vi "CoCreateGUID.vi"(8 "error in (no error)":errorcluster) -> (0 "error out":errorcluster, 2 "GUID":u8[](array[numeric]) format="%x", 4 "GUID string":string)   [LabVIEW 2017]
uses:
  ole32.dll
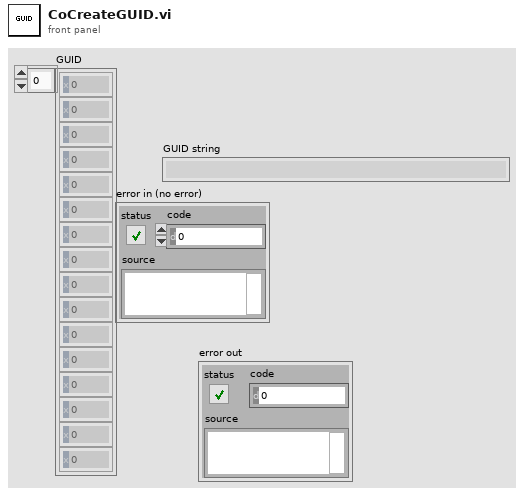
[diagram p1: front panel]
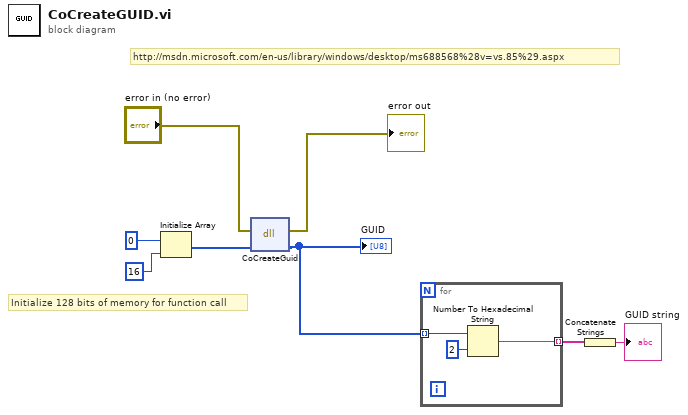
[diagram p0: block diagram]
diagram:
  # "http://msdn.microsoft.com/en-us/library/windows/desktop/ms688568%28v=vs.85%29.aspx"
  # "Initialize 128 bits of memory for function call"
  n1 = Initialize Array(u8 0 ("element"), 16 ("dimension size")) -> (w2:u8[])
  n2 = dll-call lib="ole32.dll" fn="CoCreateGuid"(error in="error in (no error)", "GUID"=w2) -> (error out=→"error out":errorcluster, "GUID"=w1:u8[])  [unwired: 3 in, 1 out]
  "GUID" <- w1
  n3 = for {
    tunnel: w1 -> [w11] mode=indexing
    tunnel: [w10] -> w6 mode=indexing
    n4 = Number To Hexadecimal String(1:i16 2 ("width (-)"), 2:w11) -> (0:w10:string)
  }
  n5 = Concatenate Strings(w6) -> (→"GUID string":string)
